vi "Cleanup.vi"(8 "error in (no error)":errorcluster, 11 "Callback Producer in":refnum<class "Callback Producer.lvclass">) -> (0 "error out":errorcluster)   [LabVIEW 2020, in "Callback Producer.lvclass"]
uses:
  Callback Producer.lvclass
  Callback Producer.lvclass/Callback Producer.ctl
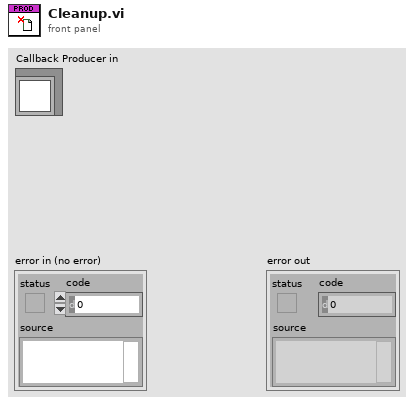
[diagram p1: front panel]
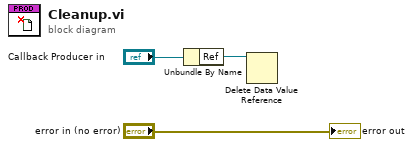
[diagram p0: block diagram]
diagram:
  n1 = Unbundle By Name("Callback Producer in") -> ("Ref"=w1:refnum<data-value>)
  n2 = Delete Data Value Reference(data value reference=w1) -> ()  [unwired: 1 in, 2 out]
  "error out" <- "error in (no error)"
